vi "axis_AcquireImage.vi"(6 "Frame Rate":u32(slide) max=30 scale=0.0..30.0, 7 "address":string="10.0.58.10", 8 "error in (no error)":errorcluster, 9 "Compression":u32(slide)=25 scale=0.0..99.0, 10 "Pixel Format":T2(ring)=enum."320 x 240 MJPG", 11 "Image In":T1) -> (0 "error out":errorcluster, 3 "Image Out":T1)   [LabVIEW 2012]
uses:
  <vilib>/vision/Image Controls.llb/IMAQ Image.ctl
panel:
  out "Content Length":i32=37577
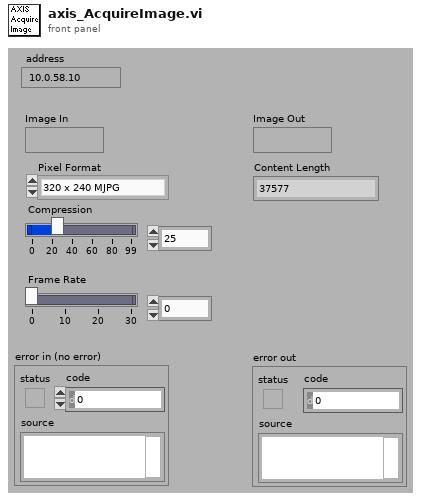
[diagram p1: front panel]
types:
  T1 = typedef "IMAQ Image.ctl" = refnum<image>
  T2 = enum16{"640 x 480 MJPG", "320 x 240 MJPG", "160 x 120 MJPG"}
  T3 = enum16{"Standard", "Buffered", "CRLF", "Immediate"}
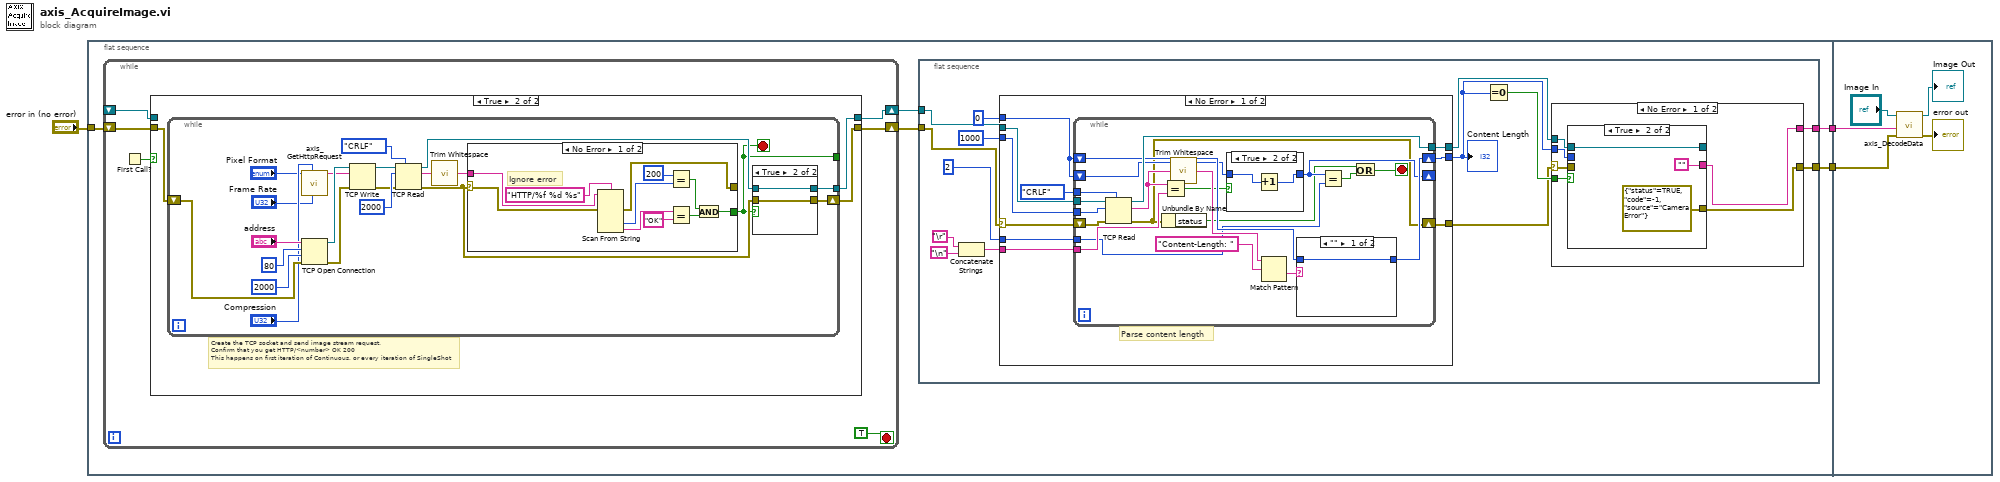
[diagram p0: block diagram]
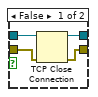
[diagram p3: hidden frame]
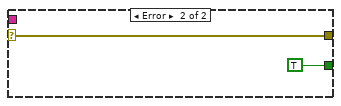
[diagram p4: hidden frame]
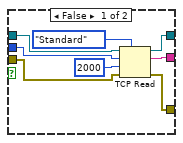
[diagram p5: hidden frame]
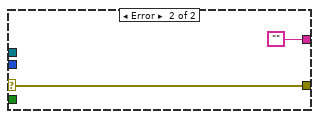
[diagram p6: hidden frame]
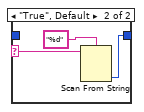
[diagram p8: hidden frame]
diagram:
  n1 = flat-sequence {
    tunnel: [w8] -> w2
    tunnel: [w4] -> w1
    tunnel: "error in (no error)" -> [w7]
    tunnel: w2 -> [w134]
    tunnel: w1 -> [w133]
    frame #0 {
      n2 = while {
        shift-right: [w11] -> w5
        shift-left: _ -> [w10]
        shift-right: [w12] -> w6
        shift-left: w7 -> [w13]
        stop <- TRUE stop-if-true
        n3 = First Call?() -> (First Call?: T/F=w9:bool)
        n4 = case shown="True" w9 {
          tunnel: w13 -> [w15 w19]
          tunnel: [w15 w18] -> w12
          tunnel: [w16 w17] -> w11
          tunnel: w10 -> [w16 _]
          frame False {
          }
          frame True {
            # "Create the TCP socket and send image stream request.\nConfirm that you get HTTP/<number> OK 200\nThis happens on first iteration of Continuous, or every iteration of SingleShot"
            n5 = while {
              shift-right: [w26] -> w18
              shift-left: w19 -> [w31]
              tunnel: [w25] -> _
              tunnel: [w27] -> w17
              stop <- w25 stop-if-true
              n6 = call "axis_GetHttpRequest.vi"("Frame Rate"="Frame Rate", "Compression"="Compression", "Pixel Format"="Pixel Format") -> ("HTTP Request"=w23:string)  [unwired: 8 out]
              n7 = TCP Open Connection(address="address", remote port or service name=u16 80, timeout ms (60000)=2000, error in (no error)=w31) -> (connection ID=w32:refnum<k5>, error out=w30:errorcluster)  [unwired: 1 out]
              n8 = TCP Write(connection ID=w32, data in=w23, error in (no error)=w30) -> (connection ID out=w36:refnum<k5>, error out=w35:errorcluster)  [unwired: 2 out]
              n9 = TCP Read(connection ID=w36, bytes to read=2000, error in (no error)=w35, 7:T3."CRLF" ("mode (standard)")) -> (connection ID out=w29:refnum<k5>, data out=w40:string, error out=w28:errorcluster)  [unwired: 1 out]
              n10 = call <vilib>:"Trim Whitespace.vi"("string"=w40) -> ("trimmed string"=w38:string)  [unwired: 1 in]
              n11 = case shown="No Error" w28 {
                selector: w28 -> [w48 w59]
                tunnel: w38 -> [w57 _]
                tunnel: [w49 TRUE] -> w25
                tunnel: [w47 w59] -> _
                frame No Error {
                  # "Ignore error"
                  n12 = Scan From String(format string="HTTP/%f %d %s", input string=w57, error in=w48) -> (error out=w47:errorcluster, output 2=w55:i32, output 3=w53:string)  [unwired: 1 in, 6 out]
                  n13 = Equal?(x=200, y=w55) -> (x = y?=w50:bool)
                  n14 = Equal?(x=w53, y="OK" ("format string")) -> (x = y?=w51:bool)
                  n15 = And(x=w50, y=w51) -> (x .and. y?=w49:bool)
                }
                frame Error {
                }
              }
              n16 = case shown="True" w25 {
                tunnel: w29 -> [w44 w46]
                tunnel: w28 -> [w43 w45]
                tunnel: [w42 w46] -> w27
                tunnel: [w41 w45] -> w26
                frame False {
                  n17 = TCP Close Connection(connection ID=w44, error in (no error)=w43) -> (connection ID out=w42:refnum<k5>, error out=w41:errorcluster)  [unwired: 1 out]
                }
                frame True {
                }
              }
            }
          }
        }
      }
      n18 = flat-sequence {
        tunnel: w6 -> [w64]
        tunnel: [w61] -> w4
        tunnel: [w63] -> w8
        tunnel: w5 -> [w62]
        frame #0 {
          n19 = Concatenate Strings("\r", "\n") -> (w73:string)
          n20 = case shown="No Error" w64 {
            selector: w64 -> [w95 w131]
            tunnel: [w102 w131] -> w67
            tunnel: [w101 w132] -> w70
            tunnel: [w100 w130] -> w69
            tunnel: w73 -> [w99 _]
            tunnel: 0 -> [w98 w132]
            tunnel: 1000 ("bytes to read") -> [w96 _]
            tunnel: w62 -> [w94 w130]
            tunnel: 2 ("y") -> [w93 _]
            frame No Error {
              # "Parse content length"
              n21 = while {
                tunnel: [w122] -> w100
                shift-right: [w118] -> w101
                shift-left: w98 -> [w117]
                shift-right: [w114] -> _
                shift-left: w98 -> [w115]
                tunnel: w99 -> [w112]
                tunnel: w96 -> [w111]
                tunnel: T3."CRLF" ("mode (standard)") -> [w110]
                shift-right: [w108] -> w102
                shift-left: w95 -> [w109]
                tunnel: w94 -> [w104]
                tunnel: w93 -> [w103]
                stop <- w105 stop-if-true
                n22 = TCP Read(connection ID=w104, bytes to read=w111, error in (no error)=w109, 7:w110) -> (connection ID out=w122:refnum<k5>, data out=w113:string, error out=w108:errorcluster)  [unwired: 1 out]
                n23 = Unbundle By Name(w108) -> ("status"=w107:bool)
                n24 = Equal?(x=w113, y=w112) -> (x = y?=w116:bool)
                n25 = call <vilib>:"Trim Whitespace.vi"("string"=w113) -> ("trimmed string"=w120:string)  [unwired: 1 in]
                n26 = case shown="True" w116 {
                  tunnel: w115 -> [w123 w125]
                  tunnel: [w123 w124] -> w114
                  frame False {
                  }
                  frame True {
                    n27 = Increment(x=w125) -> (x+1=w124:i32)
                  }
                }
                n28 = Match Pattern(string=w120, regular expression="Content-Length: ") -> (after substring=w119:string)  [unwired: 4 out]
                n29 = case shown="\"\"" w119 {
                  selector: w119 -> [_ w128]
                  tunnel: [w126 w129] -> w118
                  tunnel: w117 -> [w126 _]
                  frame "" {
                  }
                  frame "True", Default {
                    n30 = Scan From String(format string="%d", input string=w128) -> (output 1=w129:i32)  [unwired: 2 in, 4 out]
                  }
                }
                n31 = Equal?(x=w114, y=w103) -> (x = y?=w106:bool)
                n32 = Or(x=w107, y=w106) -> (x .or. y?=w105:bool)
              }
            }
            frame Error {
            }
          }
          "Content Length" <- w70
          n33 = Equal To 0?(x=w70) -> (x = 0?=w71:bool)
          n34 = case shown="No Error" w67 {
            selector: w67 -> [w74 w92]
            tunnel: [w79 w92] -> w61
            tunnel: [w78 ""] -> w63
            tunnel: w71 -> [w77 _]
            tunnel: w70 -> [w76 _]
            tunnel: w69 -> [w75 _]
            frame No Error {
              n35 = case shown="True" w77 {
                tunnel: w75 -> [w87 w89]
                tunnel: [w86 errorcluster {"status"=TRUE, "code"=-1, "source"="Camera Error"} ("error out")] -> w79
                tunnel: [w82 ""] -> w78
                tunnel: w76 -> [w83 _]
                tunnel: [w81 w89] -> _
                tunnel: w74 -> [w80 _]
                frame False {
                  n36 = TCP Read(connection ID=w87, bytes to read=w83, error in (no error)=w80, 7:T3."Standard" ("mode (standard)"), 9:2000 ("timeout ms (25000)")) -> (connection ID out=w81:refnum<k5>, data out=w82:string, error out=w86:errorcluster)
                }
                frame True {
                }
              }
            }
            frame Error {
            }
          }
        }
      }
    }
    frame #1 {
      n37 = call "axis_DecodeData.vi"("error IO"=w133, "Data In"=w134, "Image In"="Image In") -> ("error out"=→"error out":errorcluster, "Image Out"=→"Image Out":T1)  [unwired: 1 in, 6 out]
    }
  }
